vi "Rotation_Minus.vi"(9 "other ROTATION":T1={"VALUE"=0.0, "COS"=1.0, "SIN"=0.0}, 11 "in ROTATION":T1={"VALUE"=0.0, "COS"=1.0, "SIN"=0.0}) -> (3 "out ROTATION":T1)   [LabVIEW 2019, in "Trajectory_Library.lvlib"]
doc: "Subtracts the new rotation from the current rotation and returns the new rotation.\n\nFor example, Rotation2d.fromDegrees(10) - Rotation2d.fromDegrees(100) = Rotation2d{-pi/2}\n\nParameters:\n- in ROTATION - This rotation data structure\n - other ROTATION - The rotation to subtract.\n\nReturns:\n - out ROTATION - The difference between the two rotations."
uses:
  Trajectory_Library.lvlib
  ROTATION2D.ctl
  Rotation_CreateAngle.vi
  Rotation_CreateXY.vi
  Util_CalcDist.vi
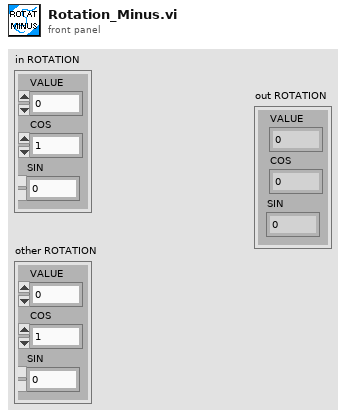
[diagram p1: front panel]
types:
  T1 = typedef "Trajectory_Library.lvlib/ROTATION2D.ctl" = cluster{"VALUE":dbl, "COS":dbl, "SIN":dbl}
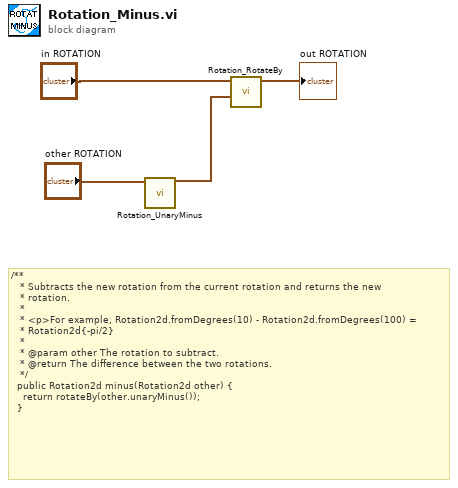
[diagram p0: block diagram]
diagram:
  # "/**\n   * Subtracts the new rotation from the current rotation and returns the new\n   * rotation.\n   *\n   * <p>For example, Rotation2d.fromDegrees(10) - Rotation2d.fromDegrees(100) =\n   * Rotation2d{-pi/2}\n   *\n   * @param other The rotation to subtract.\n   * @return The difference between the two rotations.\n   */\n  public Rotation2d minus(Rotation2d other) {\n    return rotateBy(other.unaryMinus());\n  }"
  n1 = call "Rotation_UnaryMinus.vi"("in ROTATION"="other ROTATION") -> ("out ROTATION"=w2:T1)  [unwired: 10 in]
  n2 = call "Rotation_RotateBy.vi"("other Rotation"=w2, "in ROTATION"="in ROTATION") -> ("out ROTATION"=→"out ROTATION":T1)  [unwired: 9 in]
